vi "Create GALVO Intensity Calibration File (SubVI).vi"(0 "Spot Count":i32[](array[numeric]), 6 "GALVO #":T1(ring), 8 "Image Size":T2={"Height"=3072, "Width"=3200}, 10 "Scan Spots (Array)":cluster{"X":i32, "Y":i32}[](array[cluster]), 12 "GALVO Voltage Inputs":cluster{"X":dbl, "Y ":dbl}[](array[cluster])) -> ()   [LabVIEW 2017]
uses:
  Controls (HOST)/Image Size.ctl
  <vilib>/Utility/file.llb/Write Delimited Spreadsheet (DBL).vi
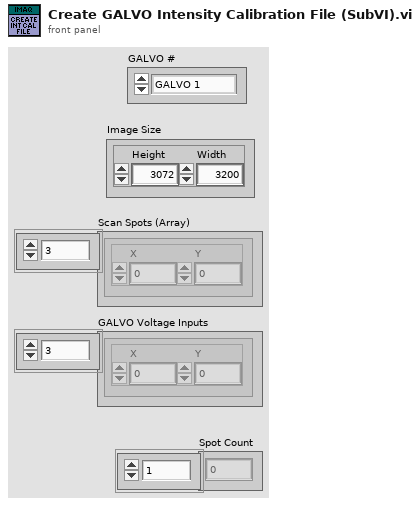
[diagram p1: front panel]
types:
  T1 = enum16{"GALVO 1", "GALVO 2", "GALVO 3", "GALVO 4"}
  T2 = typedef "Image Size.ctl" = cluster{"Height":u16, "Width":u16}
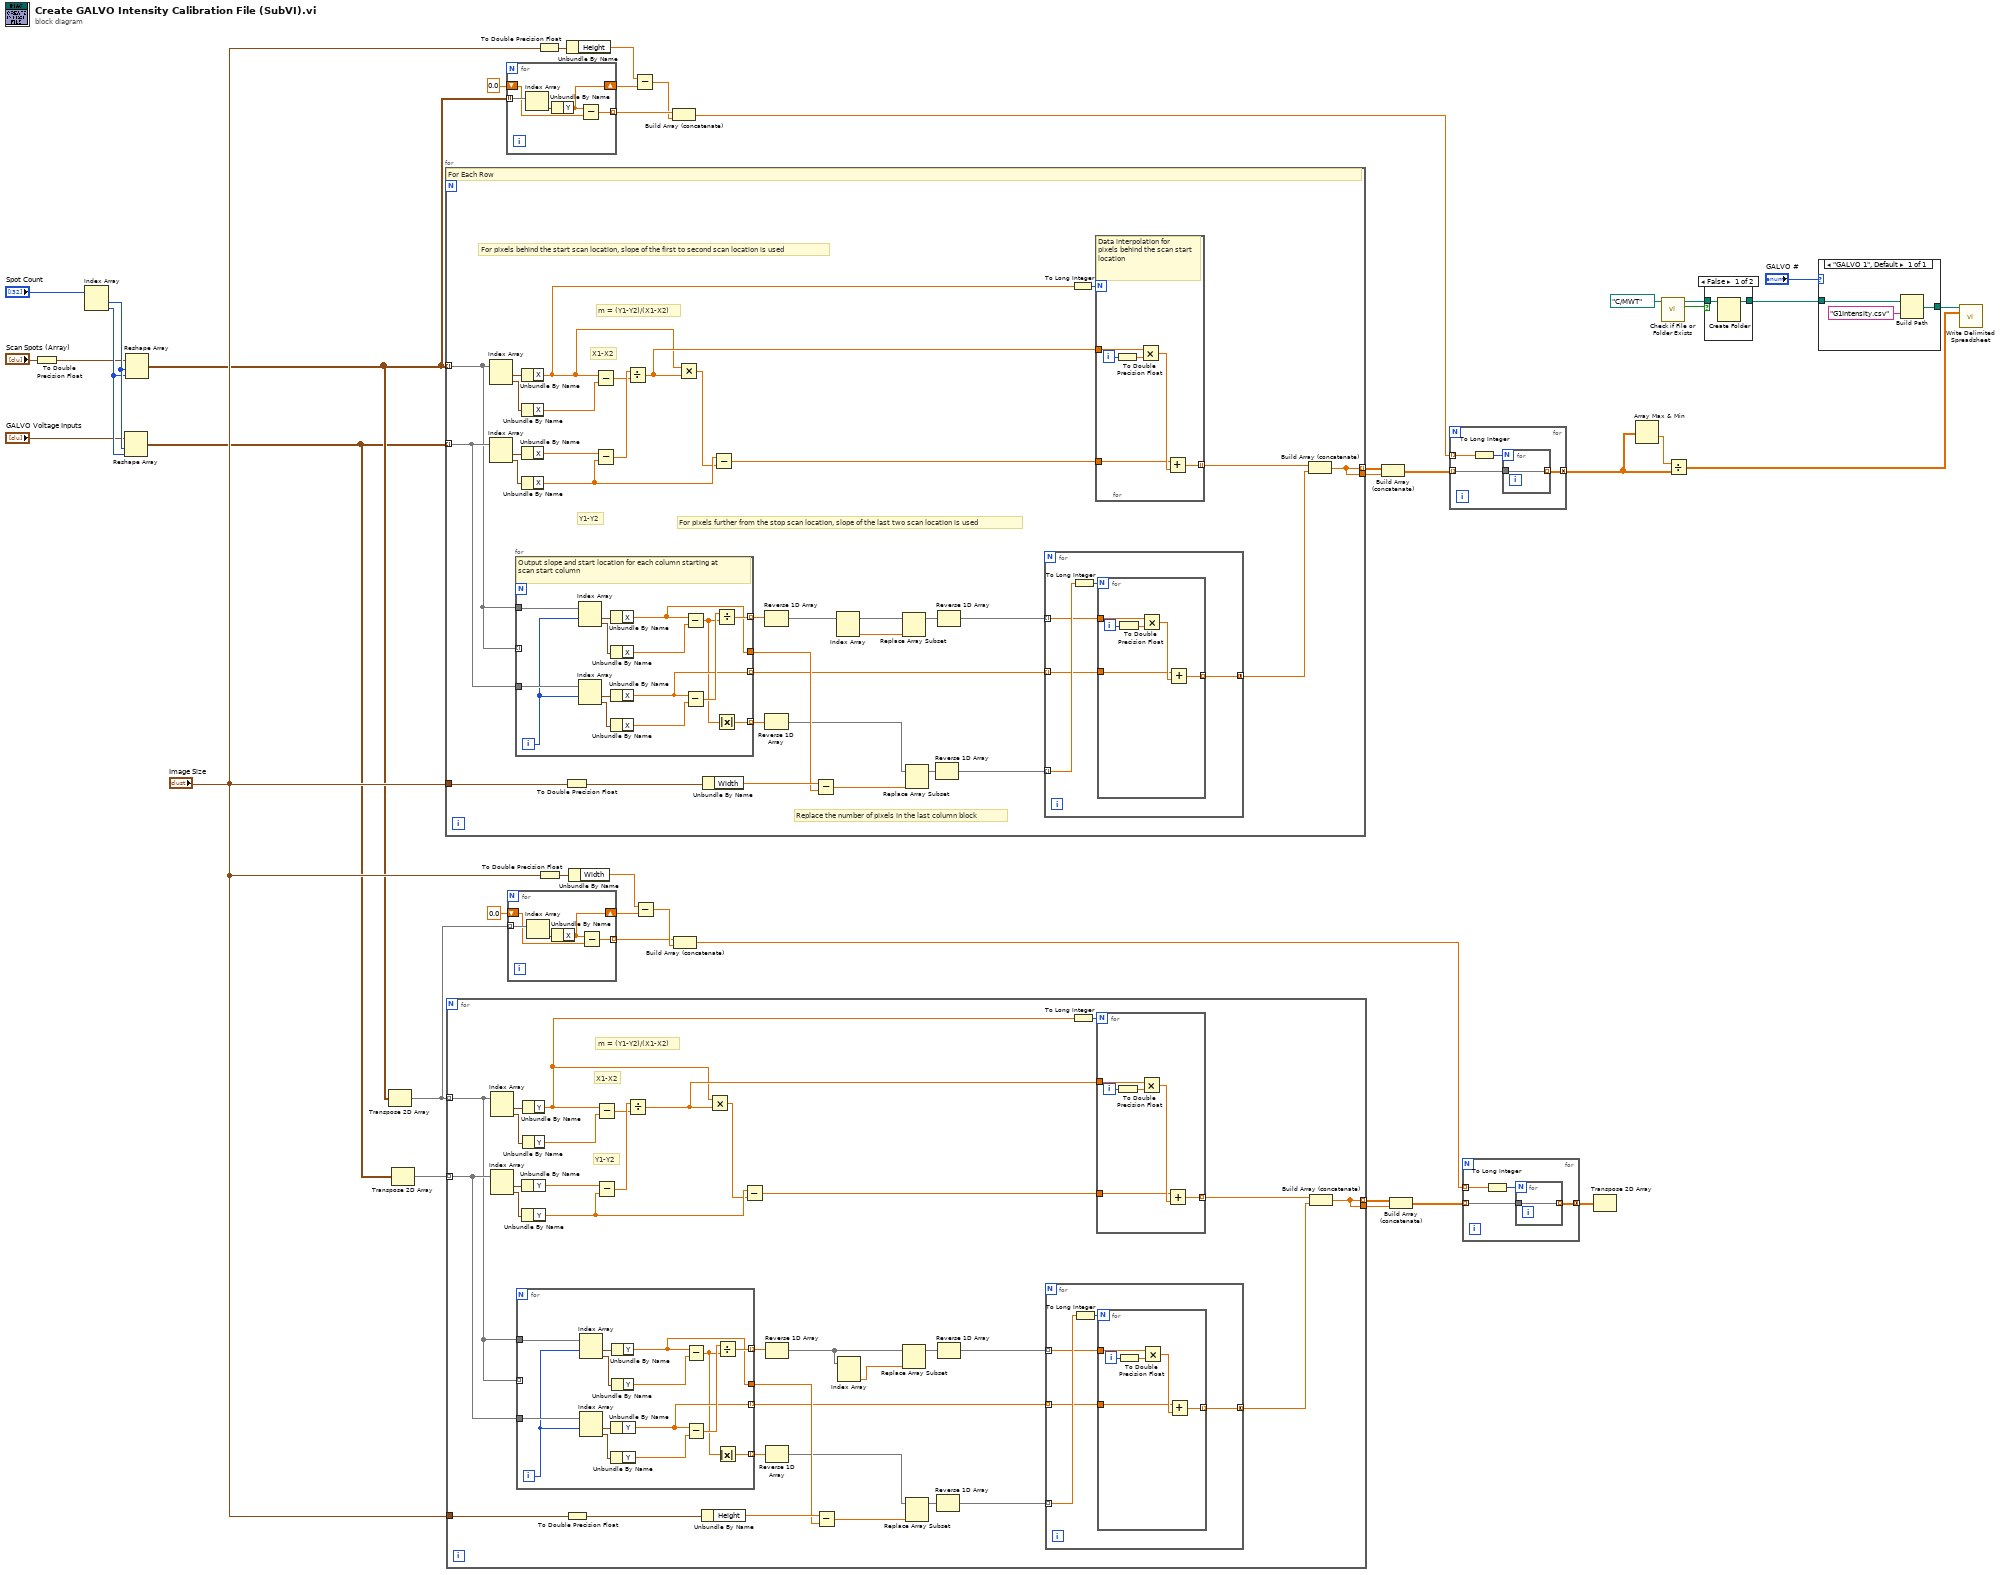
[diagram p0: block diagram]
diagram:
  n1 = To Double Precision Float(number="Scan Spots (Array)") -> (double precision float=w18:cluster{"X":dbl, "Y":dbl}[])
  n2 = Index Array(array="Spot Count") -> (element #1=w40:i32, element #2=w39:i32)  [unwired: 2 in]
  n3 = Reshape Array("GALVO Voltage Inputs", w40, w39) -> (w11:cluster{"X":dbl, "Y ":dbl}[][])
  n4 = Reshape Array(w18, w40, w39) -> (w12:cluster{"X":dbl, "Y":dbl}[][])
  n5 = Transpose 2D Array(2D array=w12) -> (transposed array=w15:cluster{"X":dbl, "Y":dbl}[][])
  n6 = Transpose 2D Array(2D array=w11) -> (transposed array=w14:cluster{"X":dbl, "Y ":dbl}[][])
  n7 = for {
    tunnel: w11 -> [w66] mode=indexing
    tunnel: w12 -> [w65] mode=indexing
    tunnel: "Image Size" -> [w62]
    tunnel: [w43] -> w10 mode=indexing
    tunnel: [w43] -> w7
    # "Replace the number of pixels in the last column block"
    # "For pixels further from the stop scan location, slope of the last two scan location is used"
    # "For pixels behind the start scan location, slope of the first to second scan location is used"
    # "m = (Y1-Y2)/(X1-X2)"
    # "X1-X2"
    # "Y1-Y2"
    # "For Each Row"
    n8 = Index Array(array=w65) -> (element #1=w75:cluster{"X":dbl, "Y":dbl}, element #2=w72:cluster{"X":dbl, "Y":dbl})  [unwired: 2 in]
    n9 = Index Array(array=w66) -> (element #1=w74:cluster{"X":dbl, "Y ":dbl}, element #2=w73:cluster{"X":dbl, "Y ":dbl})  [unwired: 2 in]
    n10 = for {
      tunnel: w65 -> [_] mode=indexing
      tunnel: w66 -> [w100]
      tunnel: w65 -> [w101]
      tunnel: [w99] -> w63 mode=indexing
      tunnel: [w98] -> w47 mode=indexing
      tunnel: [w96] -> w64 mode=indexing
      tunnel: [w93] -> w59
      i -> [w94]
      # "Output slope and start location for each column starting at scan start column"
      n11 = Index Array(array=w101, index #1=w94) -> (element #1=w102:cluster{"X":dbl, "Y":dbl}, element #2=w105:cluster{"X":dbl, "Y":dbl})  [unwired: 1 in]
      n12 = Index Array(array=w100, index #1=w94) -> (element #1=w103:cluster{"X":dbl, "Y ":dbl}, element #2=w104:cluster{"X":dbl, "Y ":dbl})  [unwired: 1 in]
      n13 = Unbundle By Name(w102) -> ("X"=w93:dbl)
      n14 = Unbundle By Name(w105) -> ("X"=w95:dbl)
      n15 = Unbundle By Name(w103) -> ("X"=w98:dbl)
      n16 = Unbundle By Name(w104) -> ("X"=w107:dbl)
      n17 = Subtract(x=w93, y=w95) -> (x-y=w97:dbl)
      n18 = Subtract(x=w98, y=w107) -> (x-y=w106:dbl)
      n19 = Divide(x=w106, y=w97) -> (x/y=w99:dbl)
      n20 = Absolute Value(x=w97) -> (abs(x)=w96:dbl)
    }
    n21 = Unbundle By Name(w75) -> ("X"=w42:dbl)
    n22 = Unbundle By Name(w72) -> ("X"=w68:dbl)
    n23 = Unbundle By Name(w74) -> ("X"=w71:dbl)
    n24 = Unbundle By Name(w73) -> ("X"=w67:dbl)
    n25 = To Double Precision Float(number=w62) -> (double precision float=w61:cluster{"Height":dbl, "Width":dbl})
    n26 = Subtract(x=w42, y=w68) -> (x-y=w69:dbl)
    n27 = Subtract(x=w71, y=w67) -> (x-y=w70:dbl)
    n28 = Divide(x=w70, y=w69) -> (x/y=w44:dbl)
    n29 = Multiply(x=w42, y=w44) -> (x*y=w51:dbl)
    n30 = Unbundle By Name(w61) -> ("Width"=w60:dbl)
    n31 = Subtract(x=w67, y=w51) -> (x-y=w50:dbl)
    n32 = Reverse 1D Array(array=w63) -> (reversed array=w58:dbl[])
    n33 = Reverse 1D Array(array=w64) -> (reversed array=w55:dbl[])
    n34 = Subtract(x=w60, y=w59) -> (x-y=w54:dbl)
    n35 = Index Array(array=w58) -> (element #2=w57:dbl)  [unwired: 2 in, 1 out]
    n36 = Replace Array Subset(array=w58, new element=w57) -> (w56:dbl[])  [unwired: 1 in]
    n37 = Replace Array Subset(array=w55, new element=w54) -> (w53:dbl[])  [unwired: 1 in]
    n38 = Reverse 1D Array(array=w53) -> (reversed array=w49:dbl[])
    n39 = Reverse 1D Array(array=w56) -> (reversed array=w48:dbl[])
    n40 = for {
      tunnel: w49 -> [w79] mode=indexing
      tunnel: [w78] -> w45 mode=concatenating
      tunnel: w48 -> [w77] mode=indexing
      tunnel: w47 -> [w76] mode=indexing
      n41 = To Long Integer(number=w79) -> (32bit integer=w80:i32)
      n42 = for {
        N: w80 -> [_]
        tunnel: w77 -> [w84]
        tunnel: w76 -> [w82]
        tunnel: [w81] -> w78 mode=indexing
        i -> [w86]
        n43 = To Double Precision Float(number=w86) -> (double precision float=w85:dbl)
        n44 = Multiply(x=w84, y=w85) -> (x*y=w83:dbl)
        n45 = Add(x=w82, y=w83) -> (x+y=w81:dbl)
      }
    }
    n46 = To Long Integer(number=w42) -> (32bit integer=w52:i32)
    n47 = for {
      N: w52 -> [_]
      tunnel: w44 -> [w90]
      tunnel: w50 -> [w88]
      tunnel: [w87] -> w46 mode=indexing
      i -> [w92]
      # "Data interpolation for pixels behind the scan start location"
      n48 = To Double Precision Float(number=w92) -> (double precision float=w91:dbl)
      n49 = Multiply(x=w90, y=w91) -> (x*y=w89:dbl)
      n50 = Add(x=w88, y=w89) -> (x+y=w87:dbl)
    }
    n51 = Build Array (concatenate)(w46, w45) -> (w43:dbl[])
  }
  n52 = for {
    tunnel: w14 -> [w132] mode=indexing
    tunnel: w15 -> [w131] mode=indexing
    tunnel: "Image Size" -> [w128]
    tunnel: [w109] -> w9 mode=indexing
    tunnel: [w109] -> w5
    # "m = (Y1-Y2)/(X1-X2)"
    # "X1-X2"
    # "Y1-Y2"
    n53 = Index Array(array=w131) -> (element #1=w141:cluster{"X":dbl, "Y":dbl}, element #2=w138:cluster{"X":dbl, "Y":dbl})  [unwired: 2 in]
    n54 = Index Array(array=w132) -> (element #1=w140:cluster{"X":dbl, "Y ":dbl}, element #2=w139:cluster{"X":dbl, "Y ":dbl})  [unwired: 2 in]
    n55 = for {
      tunnel: w131 -> [_] mode=indexing
      tunnel: w132 -> [w166]
      tunnel: w131 -> [w167]
      tunnel: [w165] -> w129 mode=indexing
      tunnel: [w164] -> w113 mode=indexing
      tunnel: [w162] -> w130 mode=indexing
      tunnel: [w159] -> w125
      i -> [w160]
      n56 = Index Array(array=w167, index #1=w160) -> (element #1=w168:cluster{"X":dbl, "Y":dbl}, element #2=w171:cluster{"X":dbl, "Y":dbl})  [unwired: 1 in]
      n57 = Index Array(array=w166, index #1=w160) -> (element #1=w169:cluster{"X":dbl, "Y ":dbl}, element #2=w170:cluster{"X":dbl, "Y ":dbl})  [unwired: 1 in]
      n58 = Unbundle By Name(w169) -> ("Y"=w164:dbl)
      n59 = Unbundle By Name(w170) -> ("Y"=w173:dbl)
      n60 = Unbundle By Name(w168) -> ("Y"=w159:dbl)
      n61 = Unbundle By Name(w171) -> ("Y"=w161:dbl)
      n62 = Subtract(x=w159, y=w161) -> (x-y=w163:dbl)
      n63 = Subtract(x=w164, y=w173) -> (x-y=w172:dbl)
      n64 = Divide(x=w172, y=w163) -> (x/y=w165:dbl)
      n65 = Absolute Value(x=w163) -> (abs(x)=w162:dbl)
    }
    n66 = Unbundle By Name(w140) -> ("Y"=w137:dbl)
    n67 = Unbundle By Name(w139) -> ("Y"=w133:dbl)
    n68 = Unbundle By Name(w141) -> ("Y"=w108:dbl)
    n69 = Unbundle By Name(w138) -> ("Y"=w134:dbl)
    n70 = To Double Precision Float(number=w128) -> (double precision float=w127:cluster{"Height":dbl, "Width":dbl})
    n71 = Subtract(x=w108, y=w134) -> (x-y=w135:dbl)
    n72 = Subtract(x=w137, y=w133) -> (x-y=w136:dbl)
    n73 = Divide(x=w136, y=w135) -> (x/y=w110:dbl)
    n74 = Unbundle By Name(w127) -> ("Height"=w126:dbl)
    n75 = Multiply(x=w108, y=w110) -> (x*y=w117:dbl)
    n76 = Subtract(x=w133, y=w117) -> (x-y=w116:dbl)
    n77 = Reverse 1D Array(array=w129) -> (reversed array=w124:dbl[])
    n78 = Reverse 1D Array(array=w130) -> (reversed array=w121:dbl[])
    n79 = Subtract(x=w126, y=w125) -> (x-y=w120:dbl)
    n80 = Index Array(array=w124) -> (element #2=w123:dbl)  [unwired: 2 in, 1 out]
    n81 = Replace Array Subset(array=w124, new element=w123) -> (w122:dbl[])  [unwired: 1 in]
    n82 = Replace Array Subset(array=w121, new element=w120) -> (w119:dbl[])  [unwired: 1 in]
    n83 = Reverse 1D Array(array=w119) -> (reversed array=w115:dbl[])
    n84 = Reverse 1D Array(array=w122) -> (reversed array=w114:dbl[])
    n85 = for {
      tunnel: w115 -> [w145] mode=indexing
      tunnel: [w144] -> w111 mode=concatenating
      tunnel: w114 -> [w143] mode=indexing
      tunnel: w113 -> [w142] mode=indexing
      n86 = To Long Integer(number=w145) -> (32bit integer=w146:i32)
      n87 = for {
        N: w146 -> [_]
        tunnel: w143 -> [w150]
        tunnel: w142 -> [w148]
        tunnel: [w147] -> w144 mode=indexing
        i -> [w152]
        n88 = To Double Precision Float(number=w152) -> (double precision float=w151:dbl)
        n89 = Multiply(x=w150, y=w151) -> (x*y=w149:dbl)
        n90 = Add(x=w148, y=w149) -> (x+y=w147:dbl)
      }
    }
    n91 = To Long Integer(number=w108) -> (32bit integer=w118:i32)
    n92 = for {
      N: w118 -> [_]
      tunnel: w110 -> [w156]
      tunnel: w116 -> [w154]
      tunnel: [w153] -> w112 mode=indexing
      i -> [w158]
      n93 = To Double Precision Float(number=w158) -> (double precision float=w157:dbl)
      n94 = Multiply(x=w156, y=w157) -> (x*y=w155:dbl)
      n95 = Add(x=w154, y=w155) -> (x+y=w153:dbl)
    }
    n96 = Build Array (concatenate)(w112, w111) -> (w109:dbl[])
  }
  n97 = for {
    tunnel: w12 -> [w178] mode=indexing
    shift-right: [w176] -> w35
    shift-left: 0.0 ("Y") -> [w175]
    tunnel: [w174] -> w34 mode=indexing
    n98 = Index Array(array=w178) -> (element=w177:cluster{"X":dbl, "Y":dbl})  [unwired: 1 in]
    n99 = Unbundle By Name(w177) -> ("Y"=w176:dbl)
    n100 = Subtract(x=w176, y=w175) -> (x-y=w174:dbl)
  }
  n101 = for {
    tunnel: w15 -> [w183] mode=indexing
    shift-right: [w181] -> w23
    shift-left: 0.0 ("Y") -> [w180]
    tunnel: [w179] -> w24 mode=indexing
    n102 = Index Array(array=w183) -> (element=w182:cluster{"X":dbl, "Y":dbl})  [unwired: 1 in]
    n103 = Unbundle By Name(w182) -> ("X"=w181:dbl)
    n104 = Subtract(x=w181, y=w180) -> (x-y=w179:dbl)
  }
  n105 = To Double Precision Float(number="Image Size") -> (double precision float=w37:cluster{"Height":dbl, "Width":dbl})
  n106 = To Double Precision Float(number="Image Size") -> (double precision float=w21:cluster{"Height":dbl, "Width":dbl})
  n107 = Unbundle By Name(w37) -> ("Height"=w36:dbl)
  n108 = Unbundle By Name(w21) -> ("Width"=w22:dbl)
  n109 = Subtract(x=w36, y=w35) -> (x-y=w33:dbl)
  n110 = Subtract(x=w22, y=w23) -> (x-y=w25:dbl)
  n111 = Build Array (concatenate)(w34, w33) -> (w32:dbl[])
  n112 = Build Array (concatenate)(w24, w25) -> (w4:dbl[])
  n113 = Build Array (concatenate)(w10, w7) -> (w8:dbl[][])
  n114 = Build Array (concatenate)(w9, w5) -> (w6:dbl[][])
  n115 = for {
    tunnel: w8 -> [w185] mode=indexing
    tunnel: w32 -> [w187] mode=indexing
    tunnel: [w184] -> w3 mode=concatenating
    n116 = To Long Integer(number=w187) -> (32bit integer=w186:i32)
    n117 = for {
      N: w186 -> [_]
      tunnel: w185 -> [w188]
      tunnel: [w188] -> w184 mode=indexing
    }
  }
  n118 = for {
    tunnel: w6 -> [w190] mode=indexing
    tunnel: w4 -> [w192] mode=indexing
    tunnel: [w189] -> w13 mode=concatenating
    n119 = To Long Integer(number=w192) -> (32bit integer=w191:i32)
    n120 = for {
      N: w191 -> [_]
      tunnel: w190 -> [w193]
      tunnel: [w193] -> w189 mode=indexing
    }
  }
  n121 = Transpose 2D Array(2D array=w13) -> ()  [unwired: 1 out]
  n122 = Array Max & Min(array=w3) -> (min value=w1:dbl)  [unwired: 3 out]
  n123 = call <vilib>:"Check if File or Folder Exists.vi"("path"=path "C:/MWT") -> ("file or folder exists?"=w29:bool, "dup path"=w30:path)  [unwired: 8 in, 1 out]
  n124 = Divide(x=w1, y=w3) -> (x/y=w2:dbl[][])
  n125 = case shown="False" w29 {
    tunnel: w30 -> [w195 w196]
    tunnel: [w194 w196] -> w26
    frame False {
      n126 = Create Folder(path (use dialog)=w195) -> (created path=w194:path)  [unwired: 2 in, 2 out]
    }
    frame True {
    }
  }
  n127 = case shown="\"GALVO 1\", Default" "GALVO #" {
    tunnel: w26 -> [w199]
    tunnel: [w197] -> w31
    frame "GALVO 1", Default {
      n128 = Build Path(base path=w199, name or relative path="G1Intensity.csv") -> (appended path=w197:path)
    }
  }
  n129 = call-poly <vilib>:"Write Delimited Spreadsheet.vi"("file path (dialog if empty)"=w31, "2D data"=w2) -> ()  [unwired: 12 in, 2 out]
